vi "Main.vi"() -> ()   [LabVIEW 2021]
doc: "This template is for the Queued Message Handler design pattern.\n\nThe Event Handling Loop generates messages based on user interface actions.\n\nThe Message Handling Loop processes messages generated by the Event Handling Loop, or by other messages. The messages are string values, so new messages can be added easily to the Message Cases case structure in the Message Handling Loop. Each message cluster can also provide an optional value for Message Data, which is a variant that can be converted to whatever message-specific data is required."
uses:
  controls/UI Data.ctl
  support/Message Queue/Enqueue Message (Single).vi
  <vilib>/Utility/error.llb/Error Cluster From Error Code.vi
  <vilib>/ErrorRing/Error Ring.xnode
  support/Message Queue/Message Queue.lvlib
  support/User Event - Stop/User Event - Stop.lvlib
panel:
  out "Logging Active":bool
  out "Log Delay":u32
  in  "Log Frequency (Hz)":dbl=2.0 min=0.0 step=0.1
  out "Sampling State":string(combo)="Paused"
  out "Pressure (bar)":dbl
  out "Pressure Chart":dbl(graph)
  out "Runtime Error out":errorcluster
  out "Measured Voltage":dbl format="%0.2f"
  out "Sample Delay mS":u32
  out "Logging State":string(combo)="Paused"
  out "Sampling Active":bool
  in  "Sample Rate (Hz)":dbl=10.0 min=0.0 step=0.1
  out "Program State":string
  in  "Start Logging":bool
  in  "Start Sampling":bool
  in  "Exit":bool
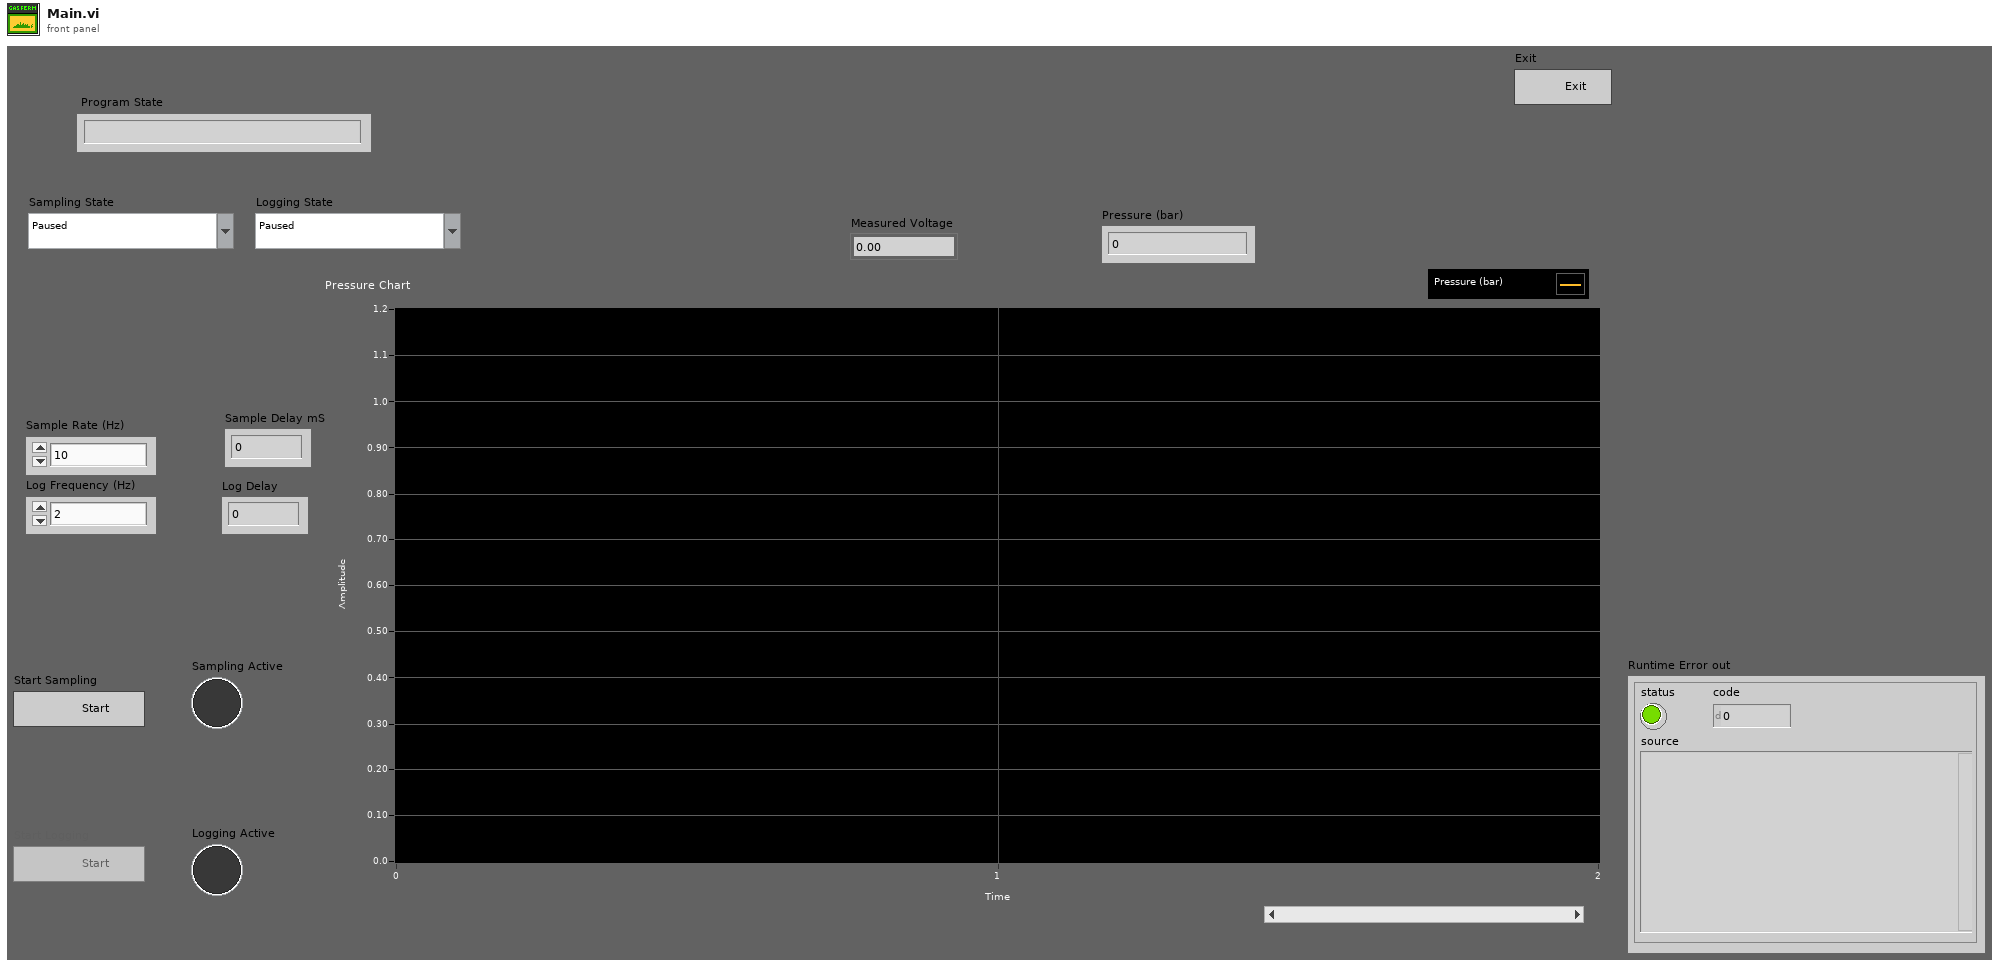
[diagram p1: front panel]
types:
  T1 = typedef "UI Data.ctl" = cluster{"Start Sampling":bool, "String <Replace Me>":string, "Numeric <Replace Me>":dbl, "Do Something Ref":refnum<vi>, "Do Something Else Ref":refnum<vi>, "Data Display Ref":refnum<vi>, "Exit Button Ref":refnum<vi>}
  T2 = typedef "Message Queue.lvlib/All Message Queues.ctl" = cluster{"UI":refnum<queue>}
  T3 = enum8{"Enabled", "Disabled", "Disabled and Grayed Out"}
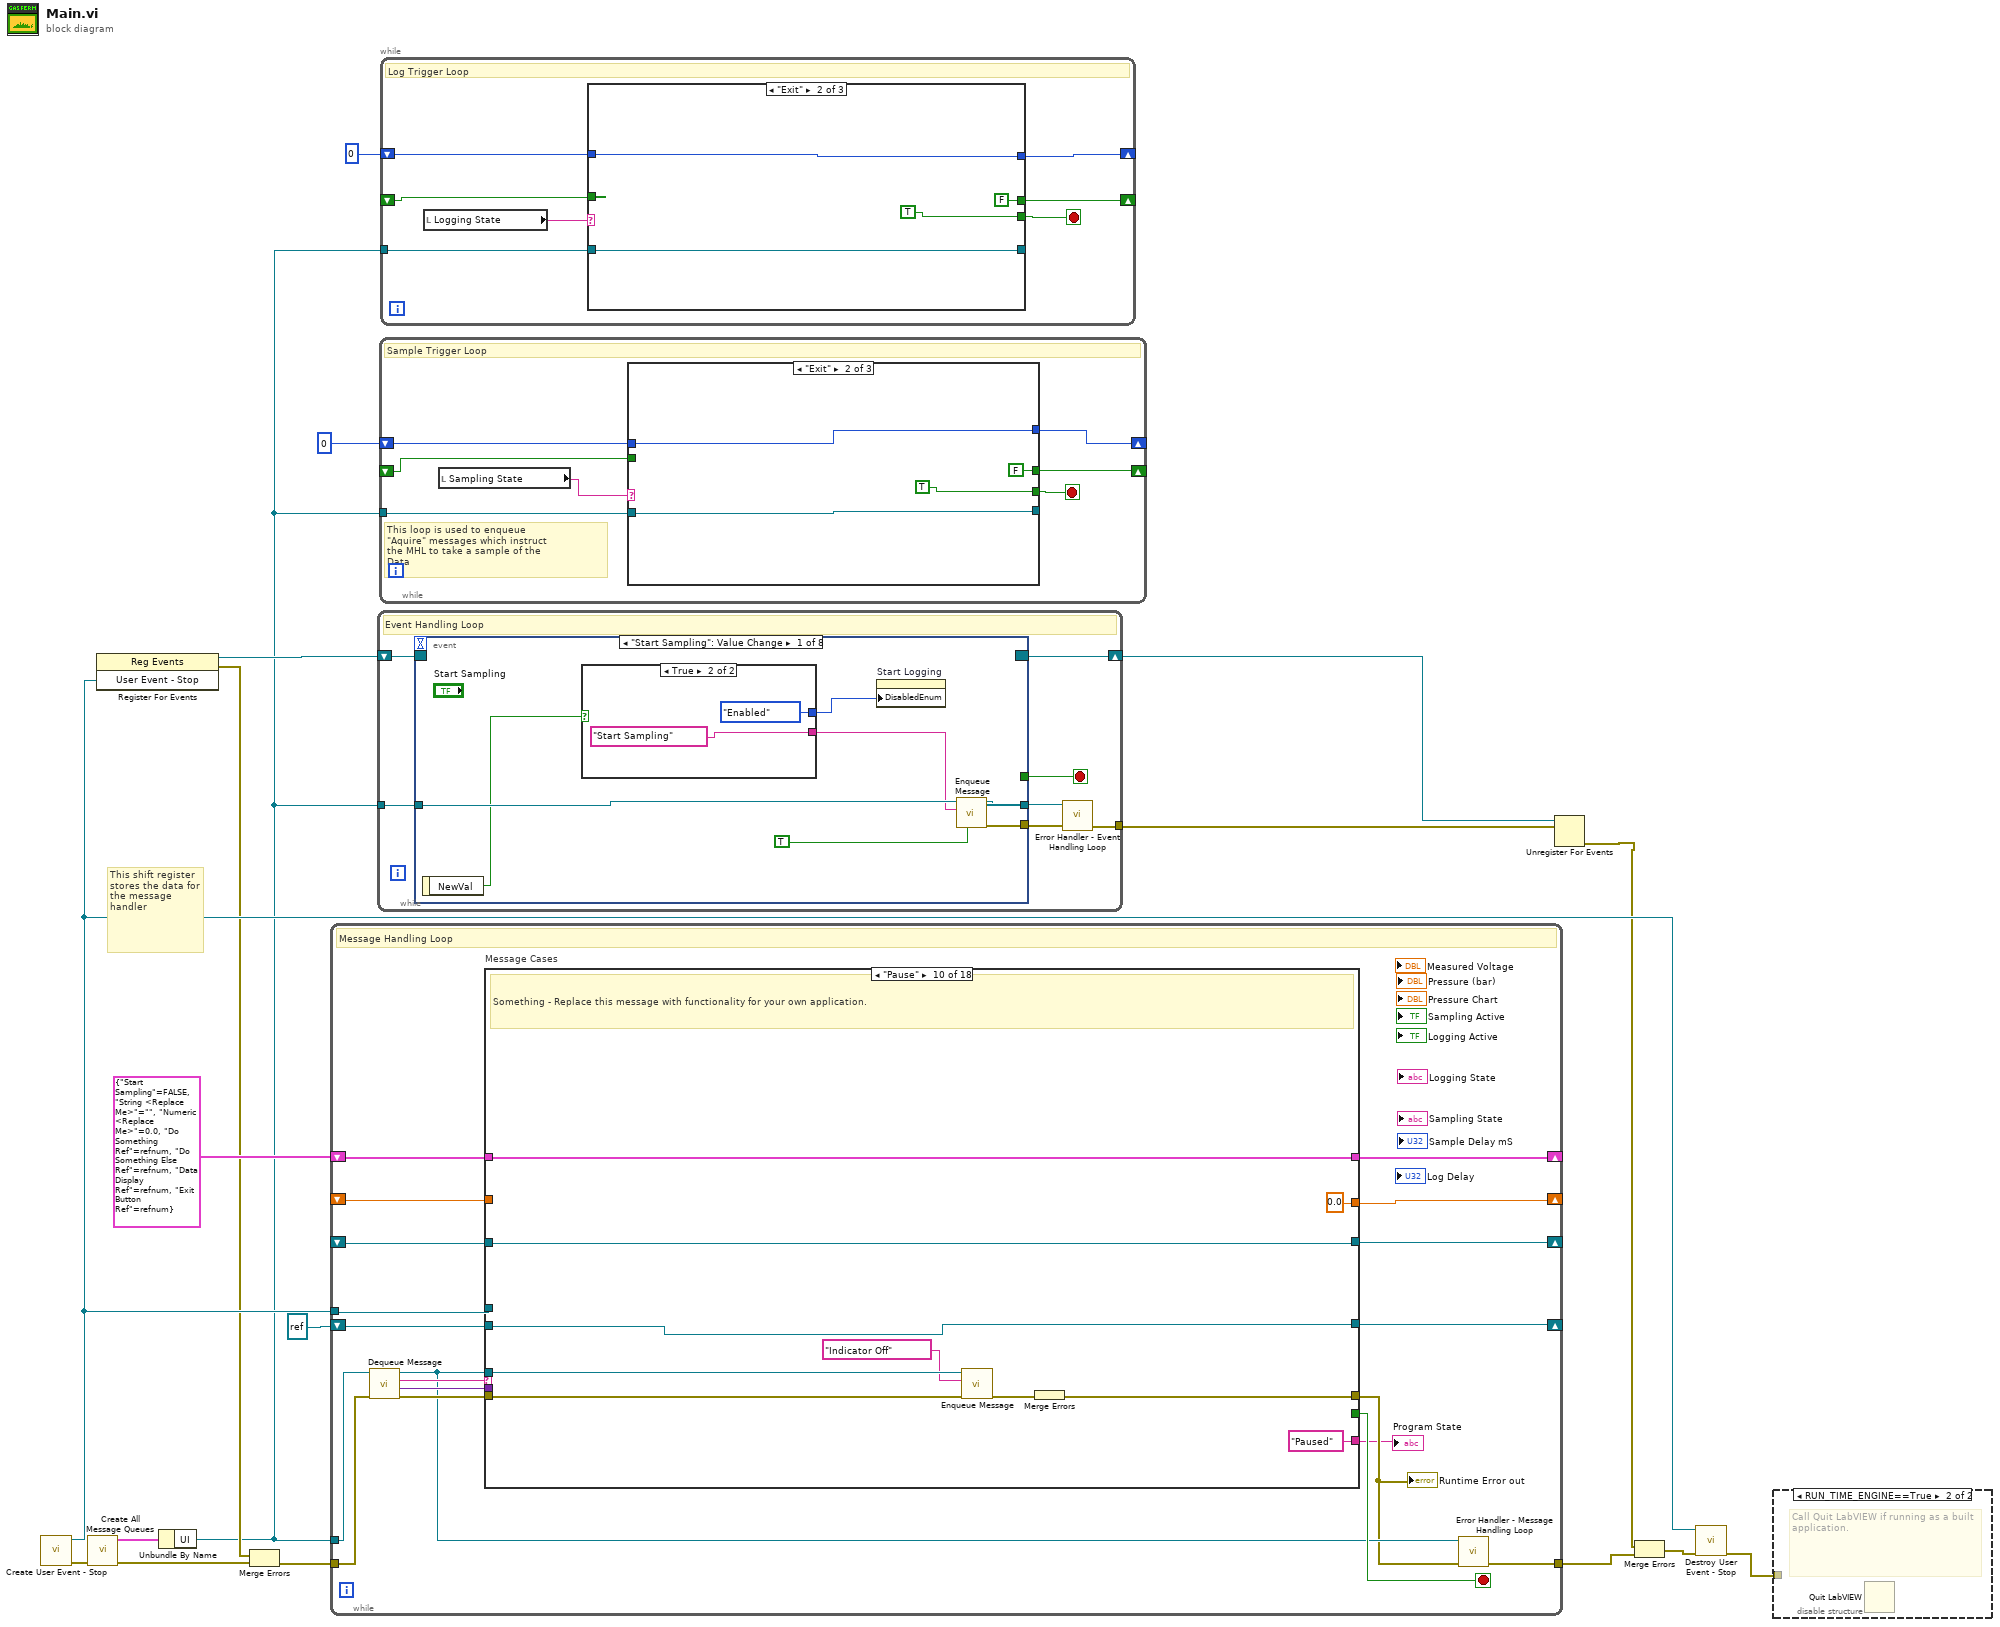
[diagram p0: block diagram]
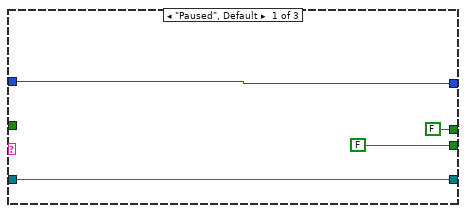
[diagram p2: hidden frame]
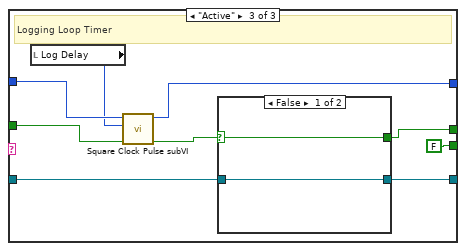
[diagram p3: hidden frame]
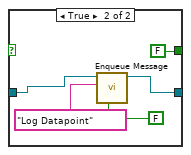
[diagram p4: hidden frame]
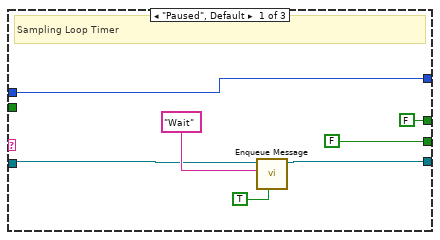
[diagram p5: hidden frame]
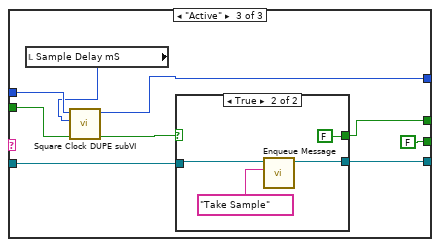
[diagram p6: hidden frame]
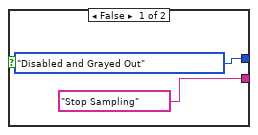
[diagram p9: hidden frame]
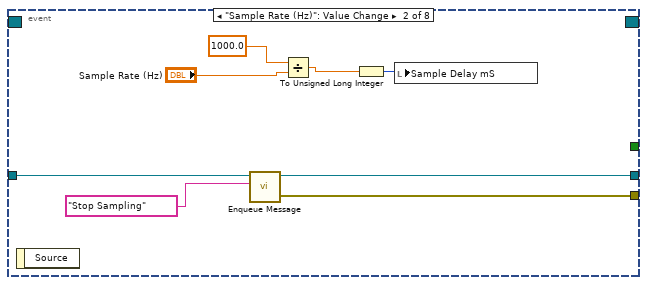
[diagram p10: hidden frame]
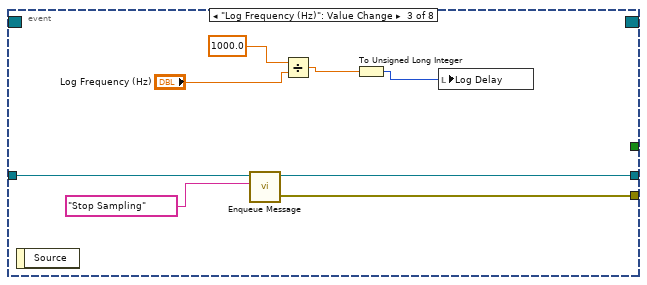
[diagram p11: hidden frame]
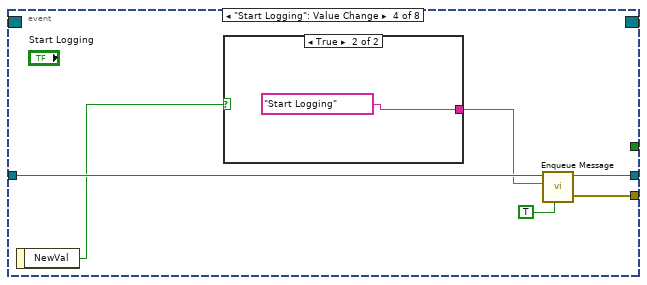
[diagram p12: hidden frame]
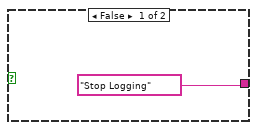
[diagram p13: hidden frame]
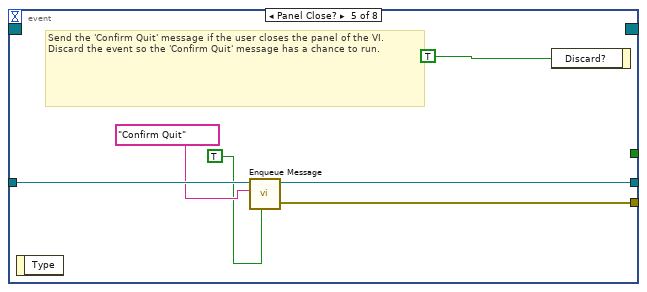
[diagram p14: hidden frame]
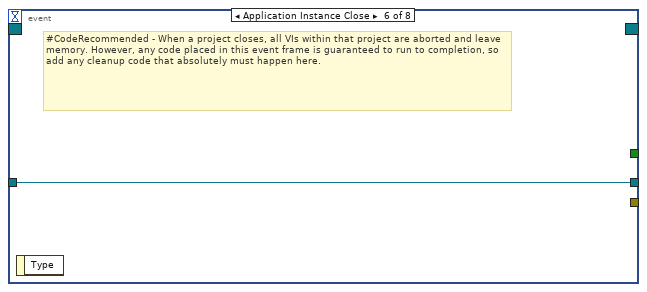
[diagram p15: hidden frame]
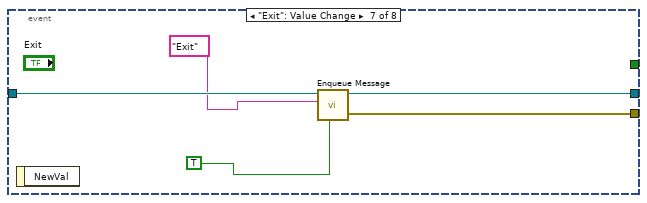
[diagram p16: hidden frame]
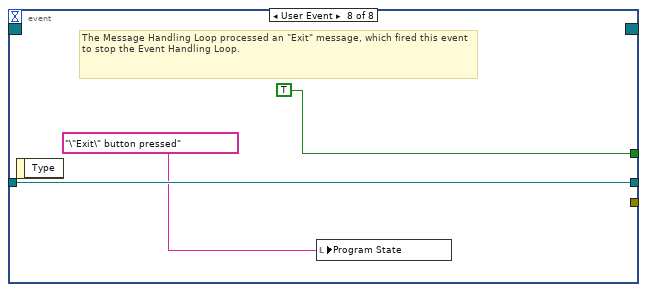
[diagram p17: hidden frame]
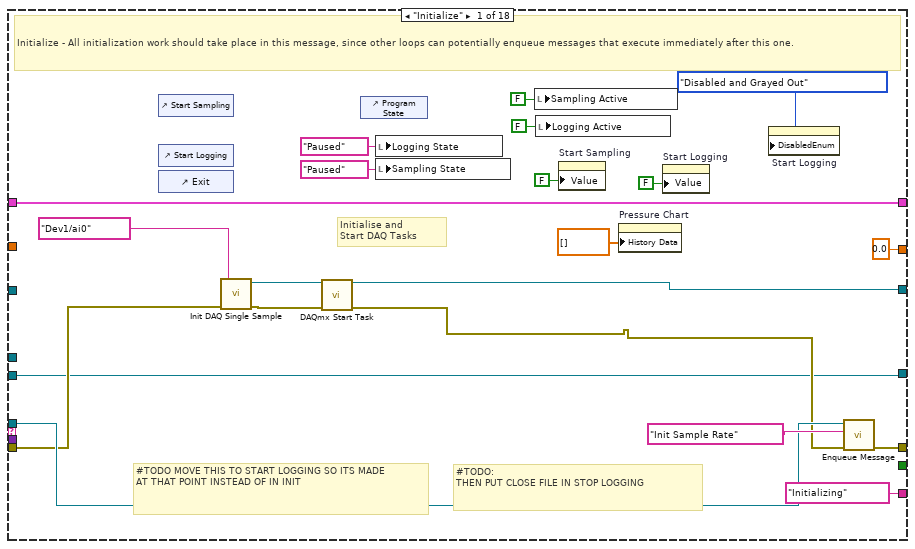
[diagram p18: hidden frame]
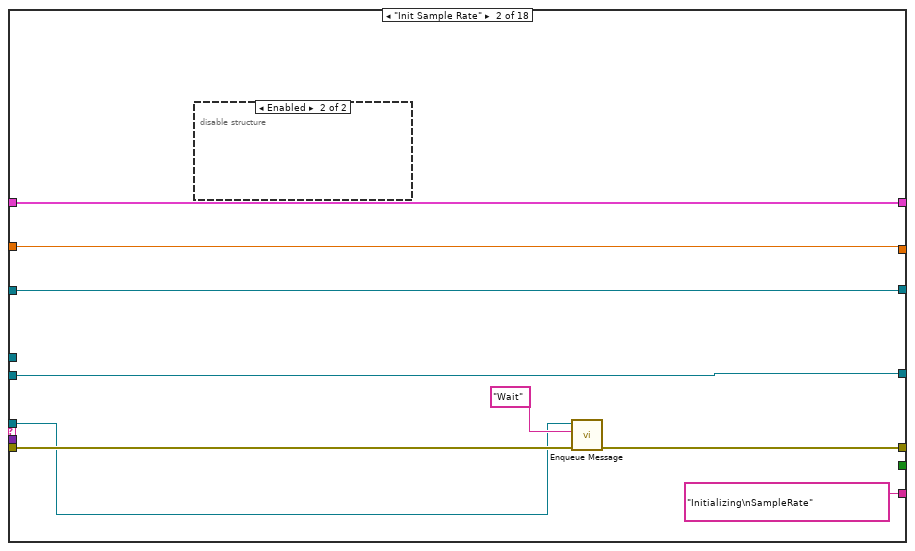
[diagram p19: hidden frame]
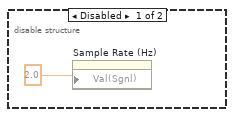
[diagram p20: hidden frame]
diagram:
  # "This shift register stores the data for the message handler"
  n1 = call "Create User Event - Stop.vi"() -> ("error out"=w16:errorcluster, "User Event - Stop"=w9:refnum<user-event>)  [unwired: 10 in]
  n2 = call "Create All Message Queues.vi"("error in (no error)"=w16) -> ("error out"=w18:errorcluster, "Message Queues out"=w17:T2)  [unwired: 9 in]
  n3 = register-events(w9) -> (reference out=w10:refnum<event-registration>, error out=w7:errorcluster)  [unwired: 2 in]
  n4 = Unbundle By Name(w17) -> ("UI"=w1:refnum<queue>)
  n5 = Merge Errors(w7, w18) -> (w8:errorcluster)
  n6 = while {
    tunnel: w1 -> [w29]
    shift-right: [w36] -> _
    shift-left: T1 {"Start Sampling"=FALSE, "String <Replace Me>"="", "Numeric <Replace Me>"=0.0, "Do Something Ref"=refnum, "Do Something Else Ref"=refnum, "Data Display Ref"=refnum, "Exit Button Ref"=refnum} ("Data Cluster") -> [w37]
    tunnel: w9 -> [w34]
    tunnel: w8 -> [w33]
    tunnel: [w27] -> w5
    shift-right: [w24] -> _
    shift-left: _ -> [w23]
    shift-right: [w22] -> _
    shift-left: refnum<file> refnum ("Byte Stream File out") -> [w21]
    shift-right: [w20] -> _
    shift-left: _ -> [w19]
    stop <- w35 stop-if-true
    # "Message Handling Loop"
    n7 = call "Dequeue Message.vi"("error in (no error)"=w33, "Message Queue"=w29) -> ("error out"=w32:errorcluster, "Message Data"=w30:variant, "Message"=w31:string, "dup Message Queue"=w28:refnum<queue>)  [unwired: 6 in]
    n8 = case "Message Cases" shown="\"Pause\"" w31 {
      selector: w31 -> [_ _ _ _ _ _ _ _ _ _ _ _ _ _ _ _ _ w268]
      tunnel: w28 -> [w56 w64 w76 w93 w103 w128 w135 w158 w174 w181 w191 w202 _ _ w234 _ w263 _]
      tunnel: w32 -> [w50 w66 w78 w95 w104 w121 w133 w154 w167 w183 w193 w204 w214 w227 w238 w245 w251 _]
      tunnel: [w58 w67 w79 w96 w109 w130 w146 w155 w171 w184 w194 w205 w215 w221 w236 w243 w259 w269] -> w26
      tunnel: w37 -> [w54 w62 w80 w97 w110 w131 w147 w159 w175 w185 w195 w206 w216 w226 w237 w244 w262 w270]
      tunnel: [w54 w62 w80 w97 w110 w131 w147 w159 w175 w185 w195 w206 w216 w226 w237 w244 w262 w270] -> w36
      tunnel: [_ _ _ _ _ _ _ _ _ _ _ _ _ _ _ _ TRUE _] -> w35
      tunnel: w30 -> [_ _ _ _ _ _ _ _ _ _ _ _ w213 w225 _ _ w254 _]
      tunnel: w34 -> [_ _ _ _ _ _ _ _ _ _ _ _ _ _ _ _ w258 _]
      tunnel: ["Initializing" "Initializing\nSampleRate" "Sampling Started" "Logging Started" "Checking State" "Logging Stopped" "Sampling Stopped" "Taking Sample" "Logging Datapoint" "Paused" "Taking Sample" "Something Else" w210 "Error Detected" "Confirming Quit" "Waiting" "Exiting" "Invalid Message"] -> w25
      tunnel: [w51 w60 w72 w89 w105 w124 w141 w153 w170 w178 w188 w197 w209 w219 w230 w241 w249 w266] -> w24
      tunnel: w23 -> [_ w60 w72 w89 w105 w124 w141 w150 w170 w178 w188 w197 w209 w219 w230 w241 w249 w266]
      tunnel: [w46 w61 w71 w83 w106 refnum<file> refnum ("Byte Stream File out") w140 w151 w168 w177 w187 w198 w208 w218 w229 w240 w248 w265] -> w22
      tunnel: w21 -> [w46 w61 w71 _ w106 w122 w140 w151 w169 w177 w187 w198 w208 w218 w229 w240 w248 w265]
      tunnel: [0.0 ("Numeric Return") w59 w70 w88 w107 w123 0.0 ("Numeric Return") w148 w164 0.0 ("Numeric Return") w186 w196 w207 w217 w228 w239 0.0 ("Numeric Return") w264] -> w20
      tunnel: w19 -> [_ w59 w70 w88 w107 w123 _ _ w165 _ w186 w196 w207 w217 w228 w239 _ w264]
      frame "Initialize" {
        # "#TODO:\nTHEN PUT CLOSE FILE IN STOP LOGGING"
        # "#TODO MOVE THIS TO START LOGGING SO ITS MADE\nAT THAT POINT INSTEAD OF IN INIT"
        # "Initialise and \nStart DAQ Tasks"
        # "Initialize - All initialization work should take place in this message, since other loops can potentially enqueue messages that execute immediately after this one."
        n9 = control-ref of="Start Sampling"() -> ()  [unwired: 1 out]
        n10 = control-ref of="Start Logging"() -> ()  [unwired: 1 out]
        n11 = control-ref of="Exit"() -> ()  [unwired: 1 out]
        n12 = call "Init DAQ Single Sample.vi"("error in"=w50, "physical channels"=tag "Dev1/ai0") -> ("error out"=w52:errorcluster, "Refnum out"=w53:refnum<k21>)  [unwired: 8 in]
        n13 = call <vilib>:"DAQmx Start Task.vi"("task/channels in"=w53, "error in"=w52) -> ("task out"=w51:refnum<k21>, "error out"=w47:errorcluster)  [unwired: 12 in]
        n14 = control-ref of="Program State"() -> ()  [unwired: 1 out]
        n15 = local write "Logging State"("Paused" ("Logging State")) -> ()
        n16 = local write "Sampling State"("Paused" ("Sampling State")) -> ()
        n17 = local write "Sampling Active"(FALSE ("Sampling Active")) -> ()
        n18 = local write "Logging Active"(FALSE ("Logging Active")) -> ()
        n19 = property on="Start Sampling" class="Bool (strict)"("Value"=FALSE ("Start Sampling")) -> ()  [unwired: 2 in, 2 out]
        n20 = property on="Pressure Chart" class="WFChart (strict)"("History Data"=dbl[] []) -> ()  [unwired: 2 in, 2 out]
        n21 = property on="Start Logging" class="Bool (strict)"("Value"=FALSE ("Start Logging")) -> ()  [unwired: 2 in, 2 out]
        n22 = property on="Start Logging" class="Bool (strict)"("DisabledEnum"=T3."Disabled and Grayed Out" ("Disabled")) -> ()  [unwired: 2 in, 2 out]
        n23 = call-poly "Enqueue Message.vi"("error in (no error)"=w47, "Message"="Init Sample Rate", "Message Queue"=w56) -> ("error out"=w58:errorcluster)  [unwired: 7 in, 1 out]
      }
      frame "Init Sample Rate" {
        n24 = disable-structure shown="Enabled" {
          frame Disabled {
            n25 = property on="Sample Rate (Hz)" class="DigNum (strict)"("Val(Sgnl)"=2.0 ("Value (Signaling)")) -> ()  [unwired: 2 in, 2 out]
          }
          frame Enabled {
          }
        }
        n26 = call-poly "Enqueue Message.vi"("error in (no error)"=w66, "Message"="Wait", "Message Queue"=w64) -> ("error out"=w67:errorcluster)  [unwired: 7 in, 1 out]
      }
      frame "Start Sampling" {
        # "Something - Replace this message with functionality for your own application."
        n27 = local write "Sampling State"("Active" ("Sampling State")) -> ()
        n28 = call-poly "Enqueue Message.vi"("error in (no error)"=w78, "Message"="Wait", "Message Queue"=w76) -> ("error out"=w77:errorcluster)  [unwired: 7 in, 1 out]
        n29 = Merge Errors(w77) -> (w79:errorcluster)
        n30 = local write "Sampling Active"(TRUE ("Sampling Active")) -> ()
      }
      frame "Start Logging" {
        w86 = "Time"  # Heading 1
        w87 = "Pressure"  # Heading 2
        w84 = "pressure-data"  # File Name
        w85 = path "Data"  # Relative Path or Folder
        # "Initialise and \nStart Log File"
        # "Something - Replace this message with functionality for your own application."
        n31 = local write "Logging Active"(TRUE ("Logging Active")) -> ()
        n32 = local write "Logging State"("Active" ("Sampling State")) -> ()
        n33 = call "Generate CSV File & Path with Headings.vi"("Heading 2"=w87, "Heading 1"=w86, "Relative Path or Folder"=w85, "File Name"=w84) -> ("error out"=w82:errorcluster, "Byte Stream File out"=w83:refnum<file>)  [unwired: 3 in, 3 out]
        n34 = call-poly "Enqueue Message.vi"("error in (no error)"=w95, "Message"="Wait", "Message Queue"=w93) -> ("error out"=w94:errorcluster)  [unwired: 7 in, 1 out]
        n35 = Merge Errors(w82, w94) -> (w96:errorcluster)
      }
      frame "Check Sampling" {
        # "Makes sure the system is in sampling mode if logging button is pressed"
        n36 = local read "Sampling State"() -> (w102:string)
        n37 = case shown="\"False\", Default" w102 {
          tunnel: w104 -> [w115 w116]
          tunnel: w103 -> [w113 w117]
          tunnel: [w112 w116] -> w101
          tunnel: [w111 w117] -> w99
          frame "False", Default {
            n38 = call-poly "Enqueue Message.vi"("error in (no error)"=w115, "Message"="Start Sampling", "Message Queue"=w113) -> ("error out"=w112:errorcluster, "dup Message Queue"=w111:refnum<queue>)  [unwired: 7 in]
          }
          frame "Active" {
          }
        }
        n39 = call-poly "Enqueue Message.vi"("error in (no error)"=w101, "Message"="Start Logging", "Message Queue"=w99) -> ("error out"=w100:errorcluster)  [unwired: 7 in, 1 out]
        n40 = Merge Errors(w100) -> (w109:errorcluster)
      }
      frame "Stop Logging" {
        # "#TODO Close Log File Here"
        # "Something - Replace this message with functionality for your own application."
        n41 = local write "Logging State"("Paused" ("Sampling State")) -> ()
        n42 = Close File(refnum=w122, error in=w121) -> (error out=w120:errorcluster)  [unwired: 1 out]
        n43 = local write "Logging Active"(FALSE ("Logging Active")) -> ()
        n44 = call-poly "Enqueue Message.vi"("error in (no error)"=w120, "Message"="Wait", "Message Queue"=w128) -> ("error out"=w129:errorcluster)  [unwired: 7 in, 1 out]
        n45 = Merge Errors(w129) -> (w130:errorcluster)
      }
      frame "Stop Sampling" {
        # "Flush Queue because too many take sample que items?"
        n46 = local write "Sampling State"("Paused" ("Sampling State")) -> ()
        n47 = local write "Logging State"("Paused" ("Sampling State")) -> ()
        n48 = Flush Queue(queue=w135, error in (no error)=w133) -> (queue out=w134:refnum<queue>, error out=w132:errorcluster)  [unwired: 1 out]
        n49 = call-poly "Enqueue Message.vi"("error in (no error)"=w132, "Message"="Wait", "Message Queue"=w134) -> ("error out"=w145:errorcluster)  [unwired: 7 in, 1 out]
        n50 = local write "Sampling Active"(FALSE ("Sampling Active")) -> ()
        n51 = local write "Logging Active"(FALSE ("Logging Active")) -> ()
        n52 = Merge Errors(w145) -> (w146:errorcluster)
      }
      frame "Take Sample" {
        # "Example use of\nformula node"
        # "Next State \nto go to here"
        # "Something - Replace this message with functionality for your own application."
        n53 = call "Take Single Sample.vi"("error in (no error)"=w154, "Refnum in"=w150) -> ("error out"=w152:errorcluster, "Voltage Detected"=w149:dbl, "Refnum out"=w153:refnum<k21>)  [unwired: 7 in]
        n54 = local write "Measured Voltage"(w149) -> ()
        n55 = formula code="Pressure= Vin / 10;"("Vin"=w149) -> ("Pressure"=w148:dbl)
        n56 = local write "Pressure Chart"(w148) -> ()
        n57 = local write "Pressure (bar)"(w148) -> ()
        n58 = call-poly "Enqueue Message.vi"("error in (no error)"=w152, "Message"="Wait", "Message Queue"=w158) -> ("error out"=w155:errorcluster)  [unwired: 7 in, 1 out]
      }
      frame "Log Datapoint" {
        # "Next State \nto go to here"
        # "Something - Replace this message with functionality for your own application."
        n59 = call "Get Current DateTime.vi"("Leading Apostrophe"=FALSE, "Use Default String"=FALSE, "Date&Time format string (%c)"="%Y_%B_%d_%H:%M.%S") -> ("Date/Time String"=w160:string)  [unwired: 5 in, 3 out]
        n60 = call "Write Numeric to CSV File.vi"("error in (no error)"=w167, "Time String"=w160, "Numeric"=w165, "Byte Stream File in"=w169) -> ("error out"=w166:errorcluster, "Numeric Return"=w164:dbl, "Byte Stream File out"=w168:refnum<file>)  [unwired: 5 in]
        n61 = call-poly "Enqueue Message.vi"("error in (no error)"=w166, "Message"="Take Sample", "Message Queue"=w174) -> ("error out"=w171:errorcluster)  [unwired: 7 in, 1 out]
      }
      frame "Pause" {
        # "Something - Replace this message with functionality for your own application."
        n62 = call-poly "Enqueue Message.vi"("error in (no error)"=w183, "Message"="Indicator Off", "Message Queue"=w181) -> ("error out"=w182:errorcluster)  [unwired: 7 in, 1 out]
        n63 = Merge Errors(w182) -> (w184:errorcluster)
      }
      frame "Indicator Off" {
        # "Something - Replace this message with functionality for your own application."
        n64 = call-poly "Enqueue Message.vi"("error in (no error)"=w193, "Message"="Wait", "Message Queue"=w191) -> ("error out"=w192:errorcluster)  [unwired: 7 in, 1 out]
        n65 = Merge Errors(w192) -> (w194:errorcluster)
      }
      frame "Something Else" {
        # "Send string to \"Update Display\" message"
        # "#CodeNeeded - Perform whatever actions correspond to the \"Something Else\" message."
        # "Something Else - Replace this message with functionality for your own application."
        n66 = call-poly "Enqueue Message.vi"("error in (no error)"=w204, "Message Data"="\"Do Something Else\" button pressed" ("\"Do Something Else\" button pressed"), "Message"="Update Display", "Message Queue"=w202) -> ("error out"=w203:errorcluster)  [unwired: 6 in, 1 out]
        n67 = Merge Errors(w203) -> (w205:errorcluster)
      }
      frame "Update Display" {
        # "#CodeRecommended - If you wish to decouple the Message Handling Loop from your user interface, consider creating User Events (like the \"Stop\" event in this VI) to message the Event Handling Loop whenever the user interface needs updating."
        # "Update Display - Convert the message data to a string to display in the Data Display indicator."
        n68 = Variant To Data(error in=w214, type="", Variant=w213) -> (data=w210:string, error out=w211:errorcluster)
        n69 = Merge Errors(w211) -> (w215:errorcluster)
      }
      frame "Error" {
        # "#CodeRecommended - If you ever change the name of this \"Error\" message, you'll need to update the name in the Check Loop Error.vi as well."
        # "#CodeRecommended - Consider creating a system for logging errors in some way. These errors are for notification purposes only. Handling of specific errors should be performed in the message frames that generated the error."
        # "Error - Display an error dialog. This message is sent by the \"Error Handler\" VIs at the end of other loops in this application."
        n70 = Variant To Data(error in=w227, type=errorcluster {"status"=FALSE, "code"=0, "source"=""} ("error constant"), Variant=w225) -> (data=w223:errorcluster, error out=w222:errorcluster)
        n71 = call <vilib>:"Simple Error Handler.vi"("error in (no error)"=w223) -> ()  [unwired: 4 in, 5 out]
        n72 = Merge Errors(w222) -> (w221:errorcluster)
      }
      frame "Confirm Quit" {
        # "#CodeNeeded - If you want to provide an \"Are you sure\" dialog (or some other notification) before the application exits, place that code here. This message is typically sent from a Panel Close? event."
        # "Confirm Quit - Message that can confirm whether or not the user wants to exit the application."
        n73 = call-poly "Enqueue Message.vi"("Priority Message? (F)"=TRUE, "error in (no error)"=w238, "Message"="Exit", "Message Queue"=w234) -> ("error out"=w235:errorcluster)  [unwired: 6 in, 1 out]
        n74 = Merge Errors(w235) -> (w236:errorcluster)
      }
      frame "Wait" {
        # "Steady State - Waiting for command from event loop or trigger loop"
        n75 = Merge Errors(w245) -> (w243:errorcluster)
      }
      frame "Exit" {
        # "Stop the VI"
        # "Release the message queue reference"
        # "#CodeNeeded - Add any required cleanup code here. Note that if 'Exit' was called as a result of an error, an error dialog will be displayed. Add any custom error handling for an 'Exit' condition here as well."
        # "Exit - Exit the application."
        n76 = Variant To Data(type=errorcluster {"status"=FALSE, "code"=0, "source"=""} ("error constant"), Variant=w254) -> (data=w255:errorcluster)  [unwired: 1 in, 1 out]
        n77 = call <vilib>:"Simple Error Handler.vi"("error in (no error)"=w255) -> ()  [unwired: 4 in, 5 out]
        n78 = call <vilib>:"DAQmx Clear Task.vi"("task in"=w249, "error in"=w251) -> ("error out"=w250:errorcluster)  [unwired: 13 in]
        n79 = call "Fire User Event - Stop.vi"("User Event - Stop"=w258) -> ("error out"=w257:errorcluster)  [unwired: 10 in]
        n80 = Release Queue(queue=w263) -> (error out=w260:errorcluster)  [unwired: 2 in, 2 out]
        n81 = Merge Errors(w257, w260, w250) -> (w259:errorcluster)
        n82 = local write "Sampling State"("Exit" ("Sampling State")) -> ()
        n83 = local write "Logging State"("Exit" ("Sampling State")) -> ()
      }
      frame Default {
        # "'Default' case only runs if there is a message that isn't defined in any of the other cases.  Output a programming error."
        n84 = xnode "Error Ring"("parameter 0"=w268) -> ("error out"=w269:errorcluster)
      }
    }
    "Program State" <- w25
    "Runtime Error out" <- w26
    n85 = call "Error Handler - Message Handling Loop.vi"("error in (no error)"=w26, "Message Queue"=w28) -> ("dup error in"=w27:errorcluster)  [unwired: 8 in, 1 out]
  }
  n86 = while {
    tunnel: w1 -> [w284]
    shift-right: [w282] -> w14
    shift-left: w10 -> [w283]
    tunnel: [w278] -> w11
    stop <- w280 stop-if-true
    # "Event Handling Loop"
    n87 = event shown="[0] \"Start Sampling\": Value Change" {
      selector: w283 -> [_ _ _ _ _ _ _ _]
      dyn-events: [_ _ _ _ _ _ _ _] -> w282
      timeout: _ -> [_ _ _ _ _ _ _ _]
      tunnel: [_ _ _ _ _ _ _ TRUE ("Discard?")] -> w280
      tunnel: w284 -> [w291 w303 w311 w317 w324 w326 w331 w334]
      tunnel: [w289 w301 w309 w315 w323 _ w330 _] -> w281
      tunnel: [w290 w302 w310 w316 w322 w326 w329 w334] -> w279
      event "Start Sampling": Value Change {
        n88 = event-data() -> ("NewVal"=w286:bool)  [unwired: 1 in]
        n89 = case shown="True" w286 {
          tunnel: ["Stop Sampling" ("Message") "Start Sampling" ("Message")] -> w288
          tunnel: [T3."Disabled and Grayed Out" ("Disabled") T3."Enabled" ("Disabled")] -> w285
          frame False {
          }
          frame True {
          }
        }
        n90 = property on="Start Logging" class="Bool (strict)"("DisabledEnum"=w285) -> ()  [unwired: 2 in, 2 out]
        n91 = call-poly "Enqueue Message.vi"("Priority Message? (F)"=TRUE, "Message"=w288, "Message Queue"=w291) -> ("error out"=w289:errorcluster, "dup Message Queue"=w290:refnum<queue>)  [unwired: 7 in]
      }
      event "Sample Rate (Hz)": Value Change {
        n92 = event-data() -> ()  [unwired: 1 in, 1 out]
        n93 = call-poly "Enqueue Message.vi"("Message"="Stop Sampling", "Message Queue"=w303) -> ("error out"=w301:errorcluster, "dup Message Queue"=w302:refnum<queue>)  [unwired: 8 in]
        n94 = Divide(x=1000.0, y="Sample Rate (Hz)") -> (x/y=w297:dbl)
        n95 = To Unsigned Long Integer(number=w297) -> (unsigned 32bit integer=w296:u32)
        n96 = local write "Sample Delay mS"(w296) -> ()
      }
      event "Log Frequency (Hz)": Value Change {
        n97 = event-data() -> ()  [unwired: 1 in, 1 out]
        n98 = call-poly "Enqueue Message.vi"("Message"="Stop Sampling", "Message Queue"=w311) -> ("error out"=w309:errorcluster, "dup Message Queue"=w310:refnum<queue>)  [unwired: 8 in]
        n99 = Divide(x=1000.0, y="Log Frequency (Hz)") -> (x/y=w306:dbl)
        n100 = To Unsigned Long Integer(number=w306) -> (unsigned 32bit integer=w304:u32)
        n101 = local write "Log Delay"(w304) -> ()
      }
      event "Start Logging": Value Change {
        n102 = event-data() -> ("NewVal"=w312:bool)  [unwired: 1 in]
        n103 = case shown="True" w312 {
          tunnel: ["Stop Logging" ("Message") "Start Logging" ("Message")] -> w314
          frame False {
          }
          frame True {
          }
        }
        n104 = call-poly "Enqueue Message.vi"("Priority Message? (F)"=TRUE, "Message"=w314, "Message Queue"=w317) -> ("error out"=w315:errorcluster, "dup Message Queue"=w316:refnum<queue>)  [unwired: 7 in]
      }
      event Panel Close? {
        # "Send the 'Confirm Quit' message if the user closes the panel of the VI. Discard the event so the 'Confirm Quit' message has a chance to run."
        n105 = event-data() -> ()  [unwired: 1 in, 1 out]
        n106 = call-poly "Enqueue Message.vi"("Priority Message? (F)"=TRUE, "Message"="Confirm Quit", "Message Queue"=w324) -> ("error out"=w323:errorcluster, "dup Message Queue"=w322:refnum<queue>)  [unwired: 7 in]
        n107 = event-data("Discard?"=TRUE) -> ()  [unwired: 1 in, 1 out]
      }
      event Application Instance Close {
        # "#CodeRecommended - When a project closes, all VIs within that project are aborted and leave memory. However, any code placed in this event frame is guaranteed to run to completion, so add any cleanup code that absolutely must happen here."
        n108 = event-data() -> ()  [unwired: 1 in, 1 out]
      }
      event "Exit": Value Change {
        n109 = event-data() -> ()  [unwired: 1 in, 1 out]
        n110 = call-poly "Enqueue Message.vi"("Priority Message? (F)"=TRUE, "Message"="Exit", "Message Queue"=w331) -> ("error out"=w330:errorcluster, "dup Message Queue"=w329:refnum<queue>)  [unwired: 7 in]
      }
      event User Event {
        # "The Message Handling Loop processed an \"Exit\" message, which fired this event to stop the Event Handling Loop."
        n111 = event-data() -> ()  [unwired: 1 in, 1 out]
        n112 = local write "Program State"("\"Exit\" button pressed" ("VI Stopped")) -> ()
      }
    }
    n113 = call "Error Handler - Event Handling Loop.vi"("error in (no error)"=w281, "Message Queue"=w279) -> ("dup error in"=w278:errorcluster)  [unwired: 8 in, 1 out]
  }
  n114 = while {
    tunnel: w1 -> [w341]
    shift-right: [w338] -> _
    shift-left: u32 0 ("Last Event mS") -> [w339]
    shift-right: [w336] -> _
    shift-left: _ -> [w335]
    stop <- w340 stop-if-true
    # "This loop is used to enqueue\n\"Aquire\" messages which instruct\nthe MHL to take a sample of the\nData"
    # "Sample Trigger Loop"
    n115 = local read "Sampling State"() -> (w337:string)
    n116 = case shown="\"Exit\"" w337 {
      tunnel: w341 -> [w345 w352 w360]
      tunnel: [w344 w352 w359] -> _
      tunnel: [FALSE TRUE FALSE] -> w340
      tunnel: w339 -> [w347 w350 w358]
      tunnel: [w347 w350 w357] -> w338
      tunnel: [FALSE FALSE w354] -> w336
      tunnel: w335 -> [_ _ w353]
      frame "Paused", Default {
        # "Sampling Loop Timer"
        n117 = call-poly "Enqueue Message.vi"("Priority Message? (F)"=TRUE, "Message"="Wait", "Message Queue"=w345) -> ("dup Message Queue"=w344:refnum<queue>)  [unwired: 7 in, 1 out]
      }
      frame "Exit" {
      }
      frame "Active" {
        n118 = local read "Sample Delay mS"() -> (w356:u32)
        n119 = call "Square Clock DUPE subVI.vi"("Last Bool State"=w353, "SampleDelay(in)"=w356, "Last Event mS"=w358) -> ("Clock Output"=w355:bool, "Last Event mS"=w357:u32)  [unwired: 5 in, 2 out]
        n120 = case shown="True" w355 {
          selector: w355 -> [w362 _]
          tunnel: w360 -> [w363 w367]
          tunnel: [w363 w366] -> w359
          tunnel: [w362 FALSE] -> w354
          frame False {
          }
          frame True {
            n121 = call-poly "Enqueue Message.vi"("Message"="Take Sample", "Message Queue"=w367) -> ("dup Message Queue"=w366:refnum<queue>)  [unwired: 8 in, 1 out]
          }
        }
      }
    }
  }
  n122 = while {
    shift-right: [w373] -> _
    shift-left: u32 0 ("Last Event mS") -> [w372]
    tunnel: w1 -> [w371]
    shift-right: [w369] -> _
    shift-left: _ -> [w368]
    stop <- w370 stop-if-true
    # "Log Trigger Loop"
    n123 = local read "Logging State"() -> (w374:string)
    n124 = case shown="\"Exit\"" w374 {
      tunnel: [w376 w380 w390] -> _
      tunnel: [FALSE TRUE FALSE] -> w370
      tunnel: [w377 w381 w387] -> w373
      tunnel: w372 -> [w377 w381 w389]
      tunnel: w371 -> [w376 w380 w386]
      tunnel: [FALSE FALSE w385] -> w369
      tunnel: w368 -> [_ _ w383]
      frame "Paused", Default {
      }
      frame "Exit" {
      }
      frame "Active" {
        # "Logging Loop Timer"
        n125 = local read "Log Delay"() -> (w384:u32)
        n126 = call "Square Clock Pulse subVI.vi"("Last Bool State"=w383, "SampleDelay(in)"=w384, "Last Event mS"=w389) -> ("Clock Output"=w388:bool, "Last Event mS"=w387:u32)  [unwired: 5 in, 2 out]
        n127 = case shown="False" w388 {
          selector: w388 -> [w392 _]
          tunnel: [w393 w398] -> w390
          tunnel: w386 -> [w393 w395]
          tunnel: [w392 FALSE] -> w385
          frame False {
          }
          frame True {
            n128 = call-poly "Enqueue Message.vi"("Priority Message? (F)"=FALSE, "Message"="Log Datapoint", "Message Queue"=w395) -> ("dup Message Queue"=w398:refnum<queue>)  [unwired: 7 in, 1 out]
          }
        }
      }
    }
  }
  n129 = Unregister For Events(event registration refnum=w14, error in=w11) -> (error out=w3:errorcluster)
  n130 = Merge Errors(w3, w5) -> (w15:errorcluster)
  n131 = call "Destroy User Event - Stop.vi"("error in (no error)"=w15, "User Event - Stop"=w9) -> ("error out"=w12:errorcluster)  [unwired: 9 in]
  n132 = disable-structure shown="RUN_TIME_ENGINE==True" {
    disable-tunnel: w12 -> [_ _]
    frame condition #0 (active) {
    }
    frame condition #1 {
      # "Call Quit LabVIEW if running as a built application."
      n133 = Quit LabVIEW() -> ()  [unwired: 1 in]
    }
  }
